vi "Read Bubble Up Working Set.vi"(8 "error in (no error)":errorcluster, 11 "Build Analyzer in":refnum<class "Build Analyzer.lvclass">) -> (0 "error out":errorcluster, 2 "Bubble Up Working Set":refnum<data-value>, 3 "Build Analyzer out":refnum<class "Build Analyzer.lvclass">)   [LabVIEW 2017, in "CL_G3_VIComponentBuilder.lvlib" / "Build Analyzer.lvclass"]
doc: "Returns the hierarchy of components in the working set as a LabVIEW Container. Given a node in the tree, the ancestors of this node are returned as dependents."
uses:
  Build Analyzer.lvclass
  <userlib>/_Cirrus Logic/LabVIEW Container/Source/Container/Container.lvclass
  Build Analyzer.lvclass/Build Analyzer.ctl
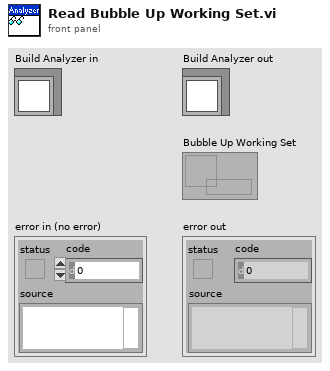
[diagram p1: front panel]
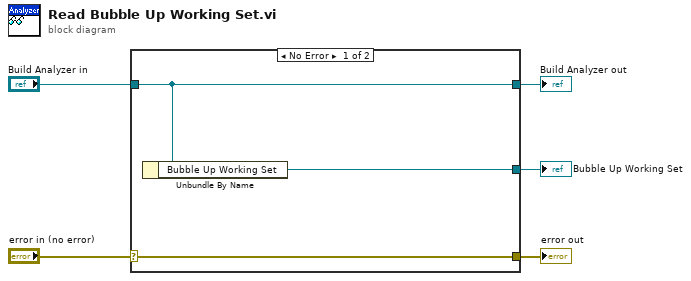
[diagram p0: block diagram]
diagram:
  n1 = case shown="No Error" "error in (no error)" {
    selector: "error in (no error)" -> [w8 w9]
    tunnel: [w8 w9] -> w4
    tunnel: [w7 w10] -> w2
    tunnel: "Build Analyzer in" -> [w7 w10]
    tunnel: [w6 _] -> w1
    frame No Error {
      n2 = Unbundle By Name(w7) -> ("Bubble Up Working Set"=w6:refnum<data-value>)
    }
    frame Error {
    }
  }
  "error out" <- w4
  "Build Analyzer out" <- w2
  "Bubble Up Working Set" <- w1
